vi "Standard Atmosphere.vi"(8 "error in (no error)":errorcluster, 11 "Altitude (m)":dbl) -> (0 "error out":errorcluster, 1 "Temperature (K)":dbl, 2 "Density (kg/m^3)":dbl, 3 "Pressure (Pa)":dbl)   [LabVIEW 2013]
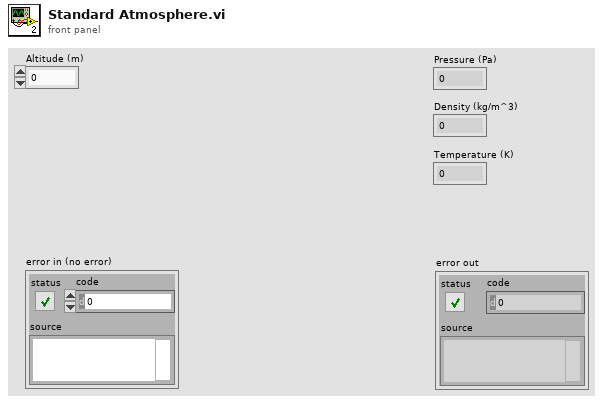
[diagram p1: front panel]
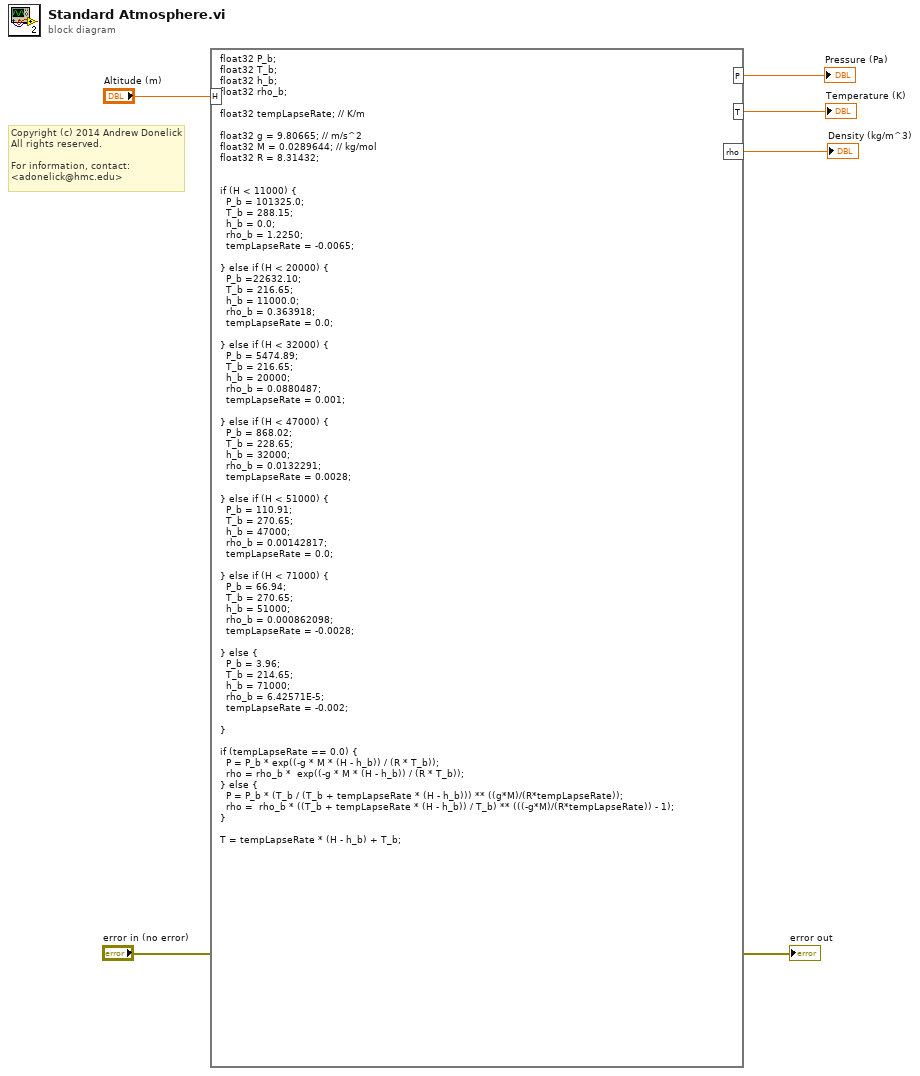
[diagram p0: block diagram]
diagram:
  # "Copyright (c) 2014 Andrew Donelick\nAll rights reserved. \n\nFor information, contact:\n<adonelick@hmc.edu>"
  n1 = formula code="float32 P_b;\nfloat32 T_b;\nfloat32 h_b;\nfloat32 rho_b;\n\nfloat32 tempLapseRate; // K/m\n\nfloat32 g = 9.80665; // m/s^2\nfloat32 M = 0.0289644; // kg/mol\nfloat32 R = 8.31432;\n\n\nif (H < 11000) {\n  P_b = 101325.0;\n  T_b = 288.15;\n  h_b = 0.0;\n  rho_b = 1.2250;\n  tempLapseRate = -0.0065;\n\n} else if (H < 20000) {\n  P_b =22632.10;\n  T_b = 216.65;\n  h_b = 11000.0;\n  rho_b = 0.363918;\n  tempLapseRate = 0.0;\n\n} else if (H < 32000) {\n  P_b = 5474.89;\n  T_b = 216.65;\n  h_b = 20000;\n  rho_b = 0.0880487;\n  tempLapseRate = 0.001;\n\n} else if (H < 47000) {\n  P_b = 868.02;\n  T_b = 228.65;\n  h_b = 32000;\n  rho_b = 0.0132291;\n  tempLapseRate = 0.0028;\n\n} else if (H < 51000) {\n  P_b = 110.91;\n  T_b = 270.65;\n  h_b = 47000;\n  rho_b = 0.00142817;\n  tempLapseRate = 0.0;\n\n} else if (H < 71000) {\n  P_b = 66.94;\n  T_b = 270.65;\n  h_b = 51000;\n  rho_b = 0.000862098;\n  tempLapseRate = -0.0028;\n\n} else {\n  P_b = 3.96;\n  T_b = 214.65;\n  h_b = 71000;\n  rho_b = 6.42571E-5;\n  tempLapseRate = -0.002;\n\n}\n\nif (tempLapseRate == 0.0) {\n  P = P_b * exp((-g * M * (H - h_b)) / (R * T_b));\n  rho = rho_b *  exp((-g * M * (H - h_b)) / (R * T_b));\n} else {\n  P = P_b * (T_b / (T_b + tempLapseRate * (H - h_b))) ** ((g*M)/(R*tempLapseRate));\n  rho =  rho_b * ((T_b + tempLapseRate * (H - h_b)) / T_b) ** (((-g*M)/(R*tempLapseRate)) - 1);\n}\n\nT = tempLapseRate * (H - h_b) + T_b;"("H"="Altitude (m)") -> ("P"=→"Pressure (Pa)":dbl, "T"=→"Temperature (K)":dbl, "rho"=→"Density (kg/m^3)":dbl)
  "error out" <- "error in (no error)"
